vi "daqcgi.vi"   [LabVIEW 2012]
doc: "This example calls a CGI that performs data acquisition. The CGI prompts the user for a channel, scan rate, and the number of samples to acquire. Once the acquisition has completed, the data is graphed on the WEB Browser.\n\nBy default this vi is in a demo mode. If you have a DAQ Board you can change the vi to non-demo mode. To change the vi to non-demo mode, change the Boolean constant in the 1shotdaq.vi labeled demo mode to false."
uses:
  <vilib>/addons/internet/NI_InternetTK_Core_VIs.lvlib
types:
  T1 = typedef "CGI Connection Info.ctl" = cluster{"name":string, "type":T2, "session":T3}
  T2 = typedef "CGI Request Type.ctl" = enum16{"cgi", ".spool first", ".spool", ".spool last"}
  T3 = typedef "HTTP Session.ctl" = refnum<k1>
  T4 = typedef "NI_FTP.lvlib/Keyed Array.ctl" = cluster{"keys":string[], "values":string[]}
  T5 = cluster{"Channel":string, "# of Scans":i32, "Scan Rate":sgl}
  T6 = typedef "Cookie.ctl" = cluster{"cookie id":string, "address":string}
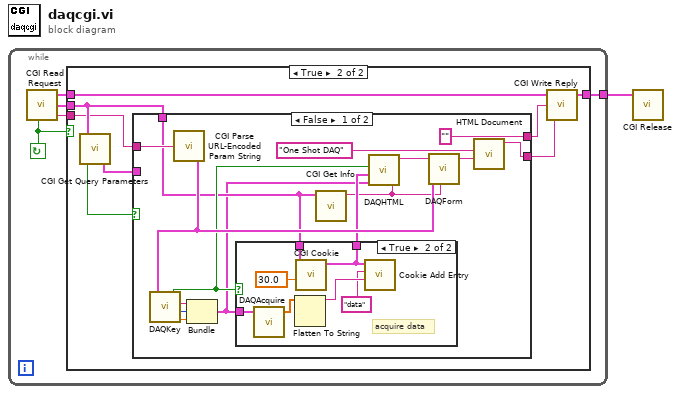
[diagram p0: block diagram]
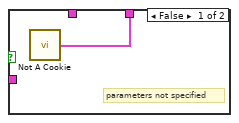
[diagram p3: hidden frame]
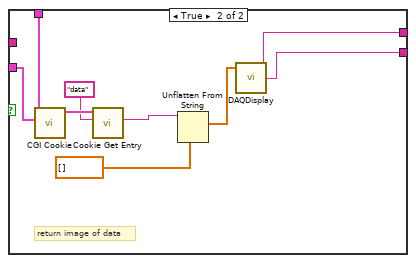
[diagram p4: hidden frame]
diagram:
  n1 = while {
    tunnel: [w5] -> w1
    stop <- w4 continue-if-true
    n2 = call <vilib>:"CGI Read Request.vi"() -> ("valid request?"=w4:bool, "cgi connection info"=w6:T1, "env"=w3:T4, "content"=w2:string)  [unwired: 4 in]
    n3 = case shown="True" w4 {
      tunnel: [w7 w15] -> w5
      tunnel: w6 -> [w7 w14]
      tunnel: w3 -> [_ w13]
      tunnel: w2 -> [_ w11]
      frame False {
      }
      frame True {
        n4 = call <vilib>:"CGI Get Query Parameters.vi"("env"=w13) -> ("query params"=w9:T4, "has query string"=w8:bool)  [unwired: 1 out]
        n5 = case shown="False" w8 {
          tunnel: w13 -> [w19 w39]
          tunnel: [w27 w46] -> w12
          tunnel: w11 -> [w26 _]
          tunnel: ["" ("header") w47] -> w10
          tunnel: w9 -> [_ w40]
          frame False {
            n6 = call <vilib>:"CGI Parse URL-Encoded Param String.vi"("url-encoded param string"=w26) -> ("params"=w24:T4)
            n7 = call "DAQKey.vi"("request"=w24) -> ("Scan Rate"=w21:sgl, "# of Scans"=w18:i32, "Channel"=w22:string, "valid"=w23:bool)  [unwired: 3 in]
            n8 = Bundle("Channel"=w22, "# of Scans"=w18, "Scan Rate"=w21) -> (w17:T5)  [unwired: 1 in]
            n9 = case shown="True" w23 {
              tunnel: [w31 w37] -> w20
              tunnel: w19 -> [_ w33]
              tunnel: w17 -> [_ w32]
              frame False {
                # "parameters not specified"
                n10 = call <vilib>:"Not A Cookie.vi"() -> ("not a cookie"=w31:T6)
              }
              frame True {
                # "acquire data"
                n11 = call "DAQAcquire.vi"("daq info"=w32) -> ("Waveform"=w38:dbl[])  [unwired: 8 in]
                n12 = Flatten To String(anything=w38) -> (data string=w35:string)  [unwired: 3 in, 2 out]
                n13 = call <vilib>:"CGI Cookie.vi"("expire time in secs (15min)"=30.0, "env"=w33) -> ("cookie"=w37:T6)  [unwired: 6 in, 3 out]
                n14 = call <vilib>:"Cookie Add Entry.vi"("value"=w35, "key"="data", "cookie"=w37) -> ()  [unwired: 1 in, 4 out]
              }
            }
            n15 = call <vilib>:"CGI Get Info.vi"("env"=w19) -> ("cgi name"=w16:string)  [unwired: 4 in, 2 out]
            n16 = call "DAQHTML.vi"("cgi name"=w16, "daq info"=w17, "cookie"=w20, "valid"=w23) -> ("HTML out"=w30:string)  [unwired: 3 in]
            n17 = call "DAQForm.vi"("HTML in"=w30, "request"=w24, "cgi name"=w16) -> ("HTML out"=w29:string)  [unwired: 6 in]
            n18 = call <vilib>:"HTML Document.vi"("document body"=w29, "document title"="One Shot DAQ") -> ("HTML Document"=w27:string)  [unwired: 9 in]
          }
          frame True {
            # "return image of data"
            n19 = call <vilib>:"CGI Cookie.vi"("params"=w40, "env"=w39) -> ("cookie"=w45:T6)  [unwired: 6 in, 3 out]
            n20 = call <vilib>:"Cookie Get Entry.vi"("key"="data", "cookie"=w45) -> ("value"=w43:string)  [unwired: 2 in, 3 out]
            n21 = Unflatten From String(type=dbl[] [] ("Waveform in"), binary string=w43) -> (value=w41:dbl[])  [unwired: 3 in, 2 out]
            n22 = call "DAQDisplay.vi"("Waveform in"=w41) -> ("header"=w47:string, "content"=w46:string)  [unwired: 7 in]
          }
        }
        n23 = call <vilib>:"CGI Write Reply.vi"("content"=w12, "header"=w10, "cgi connection info"=w14) -> ("cgi connection info out"=w15:T1)  [unwired: 2 in]
      }
    }
  }
  n24 = call <vilib>:"CGI Release.vi"("cgi connection info"=w1) -> ()  [unwired: 5 in]
